vi "simple.vi"(0 "A":dbl, 1 "B":dbl) -> (2 "Addition":dbl, 3 "Substraction":dbl, 4 "Equal":bool)   [LabVIEW 2013]
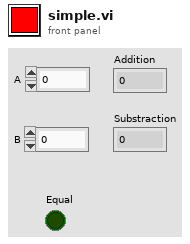
[diagram p1: front panel]
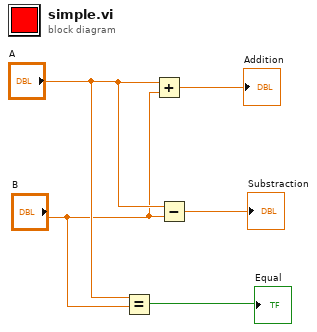
[diagram p0: block diagram]
diagram:
  n1 = Equal?(x="A", y="B") -> (x = y?=→"Equal":bool)
  n2 = Add(x="A", y="B") -> (x+y=→"Addition":dbl)
  n3 = Subtract(x="A", y="B") -> (x-y=→"Substraction":dbl)
